vi "setFont.vi"(8 "error in (no error)":errorcluster, 10 "Font":T1, 11 "Theme in":refnum<class "Theme.lvclass">) -> (0 "error out":errorcluster, 3 "Theme out":refnum<class "Theme.lvclass">)   [LabVIEW 2017, in "Theme.lvlib" / "Theme.lvclass"]
uses:
  Theme.lvclass
  Theme.Font/Font.ctl
  Theme.Font/Theme.Font.lvclass
  Theme.Font/Theme.Font.lvclass/Theme.Font.ctl
  Theme.lvclass/Theme.ctl
  Theme.Font/setSize.vi
  Theme.Font/setShrinkSize.vi
  Theme.Font/setName.vi
  Theme.Font/setPasswordDisplay.vi
  Theme.Colors/Theme.Colors.lvclass
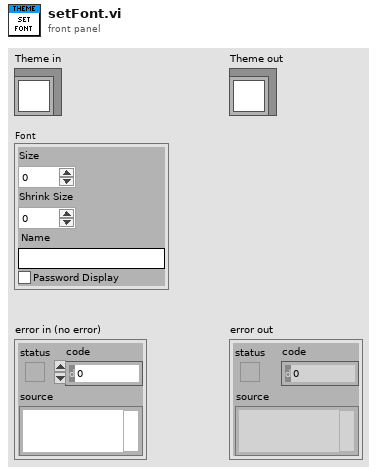
[diagram p1: front panel]
types:
  T1 = typedef "Theme.lvlib/Theme.Font.lvclass/Font.ctl" = cluster{"Size":u32, "Shrink Size":u32, "Name":string, "Password Display":bool}
  T2 = typedef "Theme.lvlib/Theme.lvclass/Private Data.ctl" = cluster{"Colors":refnum<class "Theme.Colors.lvclass">, "Font":refnum<class "Theme.Font.lvclass">}
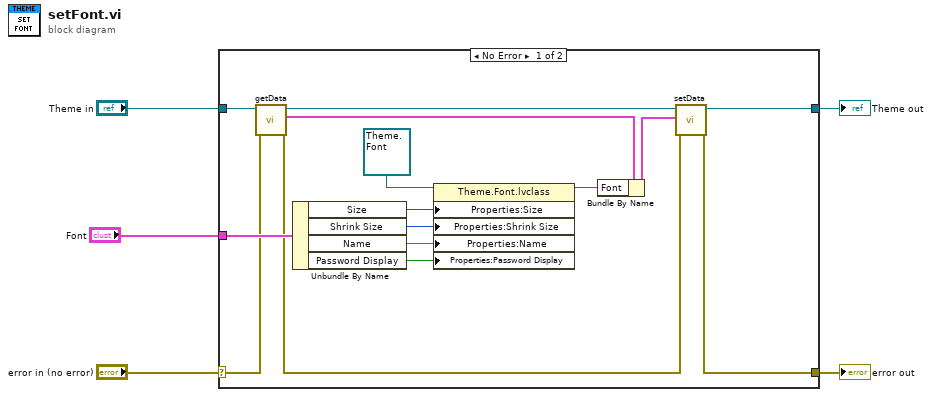
[diagram p0: block diagram]
diagram:
  n1 = case shown="No Error" "error in (no error)" {
    selector: "error in (no error)" -> [w10 w22]
    tunnel: [w8 w22] -> w4
    tunnel: [w19 w21] -> w2
    tunnel: "Theme in" -> [w18 w21]
    tunnel: "Font" -> [w14 _]
    frame No Error {
      n2 = call "getData.vi"("error in (no error)"=w10, "Theme in"=w18) -> ("error out"=w9:errorcluster, "Theme"=w17:T2, "Theme out"=w20:refnum<class "Theme.lvclass">)  [unwired: 7 in]
      n3 = Unbundle By Name(w14) -> ("Size"=w13:u32, "Shrink Size"=w12:u32, "Name"=w11:string, "Password Display"=w6:bool)
      n4 = property class="Theme.Font.lvclass"(reference=refnum<class "Theme.Font.lvclass"> refnum ("Theme.lvlib:Theme.Font.lvclass"), "Properties:Size"=w13, "Properties:Shrink Size"=w12, "Properties:Name"=w11, "Properties:Password Display"=w6) -> (reference out=w15:refnum<class "Theme.Font.lvclass">)  [unwired: 1 in, 1 out]
      n5 = Bundle By Name(cluster=w17, "Font"=w15) -> (w16:T2)
      n6 = call "setData.vi"("error in (no error)"=w9, "Theme"=w16, "Theme in"=w20) -> ("error out"=w8:errorcluster, "Theme out"=w19:refnum<class "Theme.lvclass">)  [unwired: 7 in]
    }
    frame Error {
    }
  }
  "error out" <- w4
  "Theme out" <- w2
